vi "Open Serial Comm.vi"(0 "Device ID":T1(ring), 5 "Port":i32(ring)=1 items=["COM1"=1, "COM2"=2, "COM3"=3, "COM4"=4], 7 "Interface Type":i32(ring)=70 items=["Intelligent Interface"=10, "Intelligent Interface w/ Sub"=20, "Robo Interface w/ IIM"=50, "Robo Interface"=70, "Robo Interface over RF"=80, "Robo Sub"=90, "Robo RF"=110], 11 "error in":errorcluster) -> (4 "Device ID Out":T1(ring), 15 "error out":errorcluster)   [LabVIEW 2010]
doc: "This VI opens Serial communication between your computer and the Interface Type."
uses:
  Robo Interface.dll
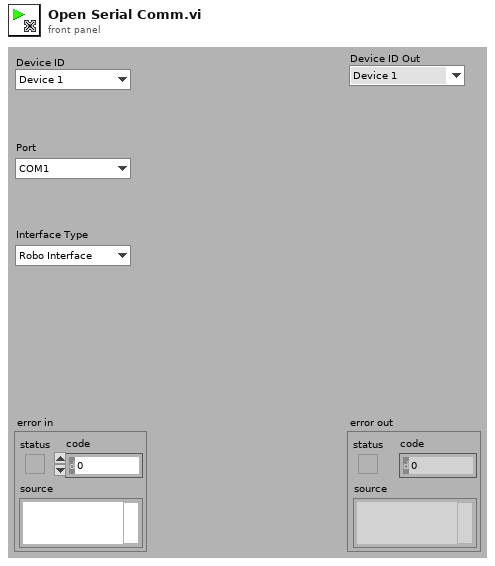
[diagram p1: front panel]
types:
  T1 = enum16{"Device 1", "Device 2", "Device 3", "Device 4", "Device 5", "Device 6", "Device 7", "Device 8"}
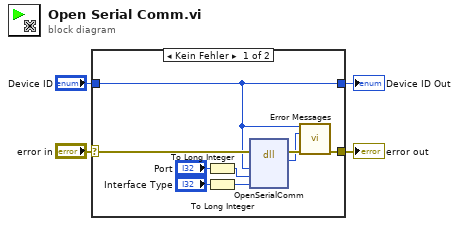
[diagram p0: block diagram]
diagram:
  n1 = case shown="Kein Fehler" "error in" {
    selector: "error in" -> [w13 w15]
    tunnel: [w11 w15] -> w3
    tunnel: "Device ID" -> [w5 w14]
    tunnel: [w5 w14] -> w1
    frame No Error {
      n2 = To Long Integer(number="Port") -> (32bit integer=w8:i32)
      n3 = To Long Integer(number="Interface Type") -> (32bit integer=w7:i32)
      n4 = dll-call lib="D:/Aron/LabVIEW-Programmierung/a.F.b.u.s.A/robo_interface_distribute/Robo Interface/Advanced/Robo Interface.dll" fn="OpenSerialComm"(error in=w13, "Device_ID"=w5, "Port"=w8, "Interface_Type"=w7) -> (error out=w12:errorcluster, "return type"=w6:i32)  [unwired: 4 in, 2 out]
      n5 = call "Error Messages.vi"("Device ID"=w5, "Error Code"=w6, "error in (no error)"=w12) -> ("error out"=w11:errorcluster)  [unwired: 12 out]
    }
    frame Error {
    }
  }
  "error out" <- w3
  "Device ID Out" <- w1
